vi "Helningsvinkel Demo.vi"() -> ()   [LabVIEW 2015]
doc: "Use this template to build a standard state machine design pattern. Each state executes code and determines which state to transition to. Contrast this design pattern with the User Interface Event Handler pattern, in which code executes in response to user actions. Contrast this design pattern also with the Queued Message Handler pattern, in which each message handling code can queue zero or more new messages."
panel:
  in  "Tab Control":T1(tab)
  in  "Senterområde \n[Grader]":dbl=10.0
  out "Horisontal":bool
  out "Calibrated Accelerations":waveform(dbl)[](graph)
  out "Helningsvinkel [Grader]":T2(graph)=[{[{"Tilt Angles [Deg][0]"=-0.6144374241661963, "Tilt Angles [Deg][1]"=86.381895519637}]}, {[{"Tilt Angles [Deg][0]"=44.252986428534086, "Tilt Angles [Deg][1]"=45.64924639869557}]}, {[{"Tilt Angles [Deg][0]"=-2.0, "Tilt Angles [Deg][1]"=-2.0}, {"Tilt Angles [Deg][0]"=-2.0, "Tilt Angles [Deg][1]"=2.0}, {"Tilt Angles [Deg][0]"=2.0, "Tilt Angles [Deg][1]"=2.0}, {"Tilt Angles [Deg][0]"=2.0, "Tilt Angles [Deg][1]"=-2.0}, {"Tilt Angles [Deg][0]"=-2.0, "Tilt Angles [Deg][1]"=-2.0}]}, {[{"Tilt Angles [Deg][0]"=90.0, "Tilt Angles [Deg][1]"=0.0}, {"Tilt Angles [Deg][0]"=87.16535433070865, "Tilt Angles [Deg][1]"=2.8346456692913384}, {"Tilt Angles [Deg][0]"=84.33070866141736, "Tilt Angles [Deg][1]"=5.669291338582677}, {"Tilt Angles [Deg][0]"=81.496062992126, "Tilt Angles [Deg][1]"=8.503937007874015}, {"Tilt Angles [Deg][0]"=78.66141732283465, "Tilt Angles [Deg][1]"=11.338582677165354}, {"Tilt Angles [Deg][0]"=75.8267716535433, "Tilt Angles [Deg][1]"=14.173228346456694}, {"Tilt Angles [Deg][0]"=72.99212598425198, "Tilt Angles [Deg][1]"=17.00787401574803}, {"Tilt Angles [Deg][0]"=70.15748031496065, "Tilt Angles [Deg][1]"=19.84251968503937}, {"Tilt Angles [Deg][0]"=67.3228346456693, "Tilt Angles [Deg][1]"=22.677165354330707}, {"Tilt Angles [Deg][0]"=64.48818897637794, "Tilt Angles [Deg][1]"=25.511811023622048}, {"Tilt Angles [Deg][0]"=61.65354330708662, "Tilt Angles [Deg][1]"=28.34645669291339}, {"Tilt Angles [Deg][0]"=58.818897637795274, "Tilt Angles [Deg][1]"=31.181102362204715}, {"Tilt Angles [Deg][0]"=55.98425196850394, "Tilt Angles [Deg][1]"=34.01574803149606}, {"Tilt Angles [Deg][0]"=53.14960629921261, "Tilt Angles [Deg][1]"=36.8503937007874}, {"Tilt Angles [Deg][0]"=50.314960629921266, "Tilt Angles [Deg][1]"=39.68503937007874}, {"Tilt Angles [Deg][0]"=47.480314960629926, "Tilt Angles [Deg][1]"=42.51968503937008}, {"Tilt Angles [Deg][0]"=44.645669291338585, "Tilt Angles [Deg][1]"=45.354330708661415}, {"Tilt Angles [Deg][0]"=41.81102362204725, "Tilt Angles [Deg][1]"=48.188976377952756}, {"Tilt Angles [Deg][0]"=38.97637795275591, "Tilt Angles [Deg][1]"=51.023622047244096}, {"Tilt Angles [Deg][0]"=36.14173228346457, "Tilt Angles [Deg][1]"=53.85826771653544}, {"Tilt Angles [Deg][0]"=33.30708661417323, "Tilt Angles [Deg][1]"=56.69291338582678}, {"Tilt Angles [Deg][0]"=30.472440944881885, "Tilt Angles [Deg][1]"=59.52755905511811}, {"Tilt Angles [Deg][0]"=27.637795275590555, "Tilt Angles [Deg][1]"=62.362204724409445}, {"Tilt Angles [Deg][0]"=24.80314960629921, "Tilt Angles [Deg][1]"=65.19685039370079}, {"Tilt Angles [Deg][0]"=21.968503937007878, "Tilt Angles [Deg][1]"=68.03149606299212}, {"Tilt Angles [Deg][0]"=19.133858267716533, "Tilt Angles [Deg][1]"=70.86614173228347}, {"Tilt Angles [Deg][0]"=16.2992125984252, "Tilt Angles [Deg][1]"=73.7007874015748}, {"Tilt Angles [Deg][0]"=13.464566929133856, "Tilt Angles [Deg][1]"=76.53543307086616}, {"Tilt Angles [Deg][0]"=10.629921259842522, "Tilt Angles [Deg][1]"=79.3700787401575}, {"Tilt Angles [Deg][0]"=7.795275590551192, "Tilt Angles [Deg][1]"=82.20472440944883}, {"Tilt Angles [Deg][0]"=4.960629921259845, "Tilt Angles [Deg][1]"=85.03937007874012}, {"Tilt Angles [Deg][0]"=2.1259842519685126, "Tilt Angles [Deg][1]"=87.8740157480315}, {"Tilt Angles [Deg][0]"=-0.7086614173228328, "Tilt Angles [Deg][1]"=89.29133858267735}, {"Tilt Angles [Deg][0]"=-3.5433070866141656, "Tilt Angles [Deg][1]"=86.45669291338587}, {"Tilt Angles [Deg][0]"=-6.377952755905511, "Tilt Angles [Deg][1]"=83.6220472440945}, {"Tilt Angles [Deg][0]"=-9.212598425196845, "Tilt Angles [Deg][1]"=80.78740157480318}, {"Tilt Angles [Deg][0]"=-12.047244094488189, "Tilt Angles [Deg][1]"=77.9527559055118}, {"Tilt Angles [Deg][0]"=-14.881889763779522, "Tilt Angles [Deg][1]"=75.11811023622049}, {"Tilt Angles [Deg][0]"=-17.716535433070867, "Tilt Angles [Deg][1]"=72.28346456692913}, {"Tilt Angles [Deg][0]"=-20.5511811023622, "Tilt Angles [Deg][1]"=69.4488188976378}, {"Tilt Angles [Deg][0]"=-23.385826771653544, "Tilt Angles [Deg][1]"=66.61417322834644}, {"Tilt Angles [Deg][0]"=-26.220472440944878, "Tilt Angles [Deg][1]"=63.77952755905513}, {"Tilt Angles [Deg][0]"=-29.05511811023622, "Tilt Angles [Deg][1]"=60.944881889763785}, {"Tilt Angles [Deg][0]"=-31.889763779527545, "Tilt Angles [Deg][1]"=58.110236220472466}, {"Tilt Angles [Deg][0]"=-34.72440944881888, "Tilt Angles [Deg][1]"=55.27559055118111}, {"Tilt Angles [Deg][0]"=-37.55905511811023, "Tilt Angles [Deg][1]"=52.44094488188977}, {"Tilt Angles [Deg][0]"=-40.393700787401585, "Tilt Angles [Deg][1]"=49.60629921259843}, {"Tilt Angles [Deg][0]"=-43.228346456692904, "Tilt Angles [Deg][1]"=46.7716535433071}, {"Tilt Angles [Deg][0]"=-46.062992125984245, "Tilt Angles [Deg][1]"=43.937007874015755}, {"Tilt Angles [Deg][0]"=-48.897637795275585, "Tilt Angles [Deg][1]"=41.102362204724415}, {"Tilt Angles [Deg][0]"=-51.73228346456693, "Tilt Angles [Deg][1]"=38.26771653543307}, {"Tilt Angles [Deg][0]"=-54.56692913385826, "Tilt Angles [Deg][1]"=35.43307086614175}, {"Tilt Angles [Deg][0]"=-57.40157480314961, "Tilt Angles [Deg][1]"=32.5984251968504}, {"Tilt Angles [Deg][0]"=-60.23622047244095, "Tilt Angles [Deg][1]"=29.763779527559056}, {"Tilt Angles [Deg][0]"=-63.070866141732296, "Tilt Angles [Deg][1]"=26.929133858267715}, {"Tilt Angles [Deg][0]"=-65.90551181102362, "Tilt Angles [Deg][1]"=24.094488188976392}, {"Tilt Angles [Deg][0]"=-68.74015748031495, "Tilt Angles [Deg][1]"=21.259842519685044}, {"Tilt Angles [Deg][0]"=-71.57480314960631, "Tilt Angles [Deg][1]"=18.4251968503937}, {"Tilt Angles [Deg][0]"=-74.40944881889763, "Tilt Angles [Deg][1]"=15.59055118110238}, {"Tilt Angles [Deg][0]"=-77.24409448818898, "Tilt Angles [Deg][1]"=12.755905511811035}, {"Tilt Angles [Deg][0]"=-80.0787401574803, "Tilt Angles [Deg][1]"=9.92125984251969}, {"Tilt Angles [Deg][0]"=-82.91338582677166, "Tilt Angles [Deg][1]"=7.0866141732283445}, {"Tilt Angles [Deg][0]"=-85.74803149606302, "Tilt Angles [Deg][1]"=4.251968503937025}, {"Tilt Angles [Deg][0]"=-88.58267716535435, "Tilt Angles [Deg][1]"=1.4173228346456799}, {"Tilt Angles [Deg][0]"=-88.58267716535435, "Tilt Angles [Deg][1]"=-1.4173228346456657}, {"Tilt Angles [Deg][0]"=-85.74803149606302, "Tilt Angles [Deg][1]"=-4.251968503937011}, {"Tilt Angles [Deg][0]"=-82.91338582677166, "Tilt Angles [Deg][1]"=-7.086614173228331}, {"Tilt Angles [Deg][0]"=-80.07874015748034, "Tilt Angles [Deg][1]"=-9.921259842519676}, {"Tilt Angles [Deg][0]"=-77.24409448818898, "Tilt Angles [Deg][1]"=-12.75590551181102}, {"Tilt Angles [Deg][0]"=-74.40944881889763, "Tilt Angles [Deg][1]"=-15.590551181102368}, {"Tilt Angles [Deg][0]"=-71.57480314960631, "Tilt Angles [Deg][1]"=-18.42519685039369}, {"Tilt Angles [Deg][0]"=-68.74015748031496, "Tilt Angles [Deg][1]"=-21.259842519685034}, {"Tilt Angles [Deg][0]"=-65.90551181102363, "Tilt Angles [Deg][1]"=-24.094488188976378}, {"Tilt Angles [Deg][0]"=-63.07086614173231, "Tilt Angles [Deg][1]"=-26.929133858267697}, {"Tilt Angles [Deg][0]"=-60.23622047244096, "Tilt Angles [Deg][1]"=-29.763779527559045}, {"Tilt Angles [Deg][0]"=-57.401574803149614, "Tilt Angles [Deg][1]"=-32.598425196850386}, {"Tilt Angles [Deg][0]"=-54.56692913385827, "Tilt Angles [Deg][1]"=-35.43307086614173}, {"Tilt Angles [Deg][0]"=-51.732283464566954, "Tilt Angles [Deg][1]"=-38.26771653543305}, {"Tilt Angles [Deg][0]"=-48.89763779527561, "Tilt Angles [Deg][1]"=-41.1023622047244}, {"Tilt Angles [Deg][0]"=-46.06299212598426, "Tilt Angles [Deg][1]"=-43.93700787401575}, {"Tilt Angles [Deg][0]"=-43.22834645669291, "Tilt Angles [Deg][1]"=-46.77165354330708}, {"Tilt Angles [Deg][0]"=-40.39370078740159, "Tilt Angles [Deg][1]"=-49.60629921259841}, {"Tilt Angles [Deg][0]"=-37.55905511811025, "Tilt Angles [Deg][1]"=-52.440944881889756}, {"Tilt Angles [Deg][0]"=-34.724409448818896, "Tilt Angles [Deg][1]"=-55.275590551181104}, {"Tilt Angles [Deg][0]"=-31.88976377952756, "Tilt Angles [Deg][1]"=-58.11023622047245}, {"Tilt Angles [Deg][0]"=-29.055118110236215, "Tilt Angles [Deg][1]"=-60.944881889763785}, {"Tilt Angles [Deg][0]"=-26.220472440944917, "Tilt Angles [Deg][1]"=-63.77952755905508}, {"Tilt Angles [Deg][0]"=-23.38582677165357, "Tilt Angles [Deg][1]"=-66.61417322834644}, {"Tilt Angles [Deg][0]"=-20.55118110236223, "Tilt Angles [Deg][1]"=-69.44881889763776}, {"Tilt Angles [Deg][0]"=-17.71653543307088, "Tilt Angles [Deg][1]"=-72.28346456692913}, {"Tilt Angles [Deg][0]"=-14.881889763779538, "Tilt Angles [Deg][1]"=-75.11811023622046}, {"Tilt Angles [Deg][0]"=-12.047244094488189, "Tilt Angles [Deg][1]"=-77.9527559055118}, {"Tilt Angles [Deg][0]"=-9.212598425196845, "Tilt Angles [Deg][1]"=-80.78740157480314}, {"Tilt Angles [Deg][0]"=-6.3779527559055005, "Tilt Angles [Deg][1]"=-83.6220472440945}, {"Tilt Angles [Deg][0]"=-3.543307086614205, "Tilt Angles [Deg][1]"=-86.45669291338577}, {"Tilt Angles [Deg][0]"=-0.7086614173228596, "Tilt Angles [Deg][1]"=-89.29133858267735}, {"Tilt Angles [Deg][0]"=2.125984251968486, "Tilt Angles [Deg][1]"=-87.8740157480315}, {"Tilt Angles [Deg][0]"=4.96062992125983, "Tilt Angles [Deg][1]"=-85.03937007874019}, {"Tilt Angles [Deg][0]"=7.795275590551176, "Tilt Angles [Deg][1]"=-82.20472440944883}, {"Tilt Angles [Deg][0]"=10.629921259842522, "Tilt Angles [Deg][1]"=-79.3700787401575}, {"Tilt Angles [Deg][0]"=13.464566929133868, "Tilt Angles [Deg][1]"=-76.53543307086613}, {"Tilt Angles [Deg][0]"=16.299212598425164, "Tilt Angles [Deg][1]"=-73.70078740157484}, {"Tilt Angles [Deg][0]"=19.133858267716505, "Tilt Angles [Deg][1]"=-70.8661417322835}, {"Tilt Angles [Deg][0]"=21.968503937007853, "Tilt Angles [Deg][1]"=-68.03149606299215}, {"Tilt Angles [Deg][0]"=24.803149606299197, "Tilt Angles [Deg][1]"=-65.1968503937008}, {"Tilt Angles [Deg][0]"=27.63779527559054, "Tilt Angles [Deg][1]"=-62.36220472440946}, {"Tilt Angles [Deg][0]"=30.472440944881885, "Tilt Angles [Deg][1]"=-59.52755905511811}, {"Tilt Angles [Deg][0]"=33.30708661417324, "Tilt Angles [Deg][1]"=-56.69291338582678}, {"Tilt Angles [Deg][0]"=36.14173228346458, "Tilt Angles [Deg][1]"=-53.85826771653543}, {"Tilt Angles [Deg][0]"=38.976377952755875, "Tilt Angles [Deg][1]"=-51.023622047244125}, {"Tilt Angles [Deg][0]"=41.811023622047216, "Tilt Angles [Deg][1]"=-48.18897637795279}, {"Tilt Angles [Deg][0]"=44.645669291338564, "Tilt Angles [Deg][1]"=-45.35433070866144}, {"Tilt Angles [Deg][0]"=47.480314960629904, "Tilt Angles [Deg][1]"=-42.519685039370096}, {"Tilt Angles [Deg][0]"=50.31496062992125, "Tilt Angles [Deg][1]"=-39.685039370078755}, {"Tilt Angles [Deg][0]"=53.1496062992126, "Tilt Angles [Deg][1]"=-36.8503937007874}, {"Tilt Angles [Deg][0]"=55.98425196850395, "Tilt Angles [Deg][1]"=-34.01574803149605}, {"Tilt Angles [Deg][0]"=58.81889763779525, "Tilt Angles [Deg][1]"=-31.18110236220476}, {"Tilt Angles [Deg][0]"=61.653543307086586, "Tilt Angles [Deg][1]"=-28.346456692913417}, {"Tilt Angles [Deg][0]"=64.48818897637793, "Tilt Angles [Deg][1]"=-25.511811023622073}, {"Tilt Angles [Deg][0]"=67.32283464566927, "Tilt Angles [Deg][1]"=-22.67716535433073}, {"Tilt Angles [Deg][0]"=70.15748031496062, "Tilt Angles [Deg][1]"=-19.84251968503938}, {"Tilt Angles [Deg][0]"=72.99212598425198, "Tilt Angles [Deg][1]"=-17.007874015748037}, {"Tilt Angles [Deg][0]"=75.82677165354332, "Tilt Angles [Deg][1]"=-14.17322834645669}, {"Tilt Angles [Deg][0]"=78.66141732283465, "Tilt Angles [Deg][1]"=-11.338582677165345}, {"Tilt Angles [Deg][0]"=81.49606299212596, "Tilt Angles [Deg][1]"=-8.50393700787405}, {"Tilt Angles [Deg][0]"=84.33070866141729, "Tilt Angles [Deg][1]"=-5.669291338582704}, {"Tilt Angles [Deg][0]"=87.16535433070865, "Tilt Angles [Deg][1]"=-2.8346456692913593}, {"Tilt Angles [Deg][0]"=90.0, "Tilt Angles [Deg][1]"=-1.4033418597069752e-14}]}]
  # "Helningsmåling med akselerometer"
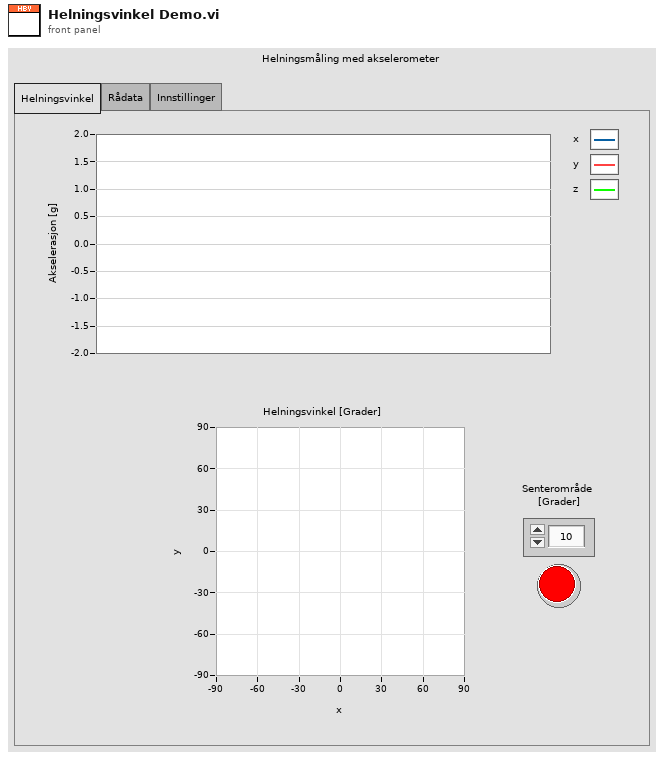
[diagram p1: front panel]
types:
  T1 = enum32{"Helningsvinkel", "Rådata", "Innstillinger"}
  T2 = cluster{cluster{"Tilt Angles [Deg][0]":dbl, "Tilt Angles [Deg][1]":dbl}[]}[]
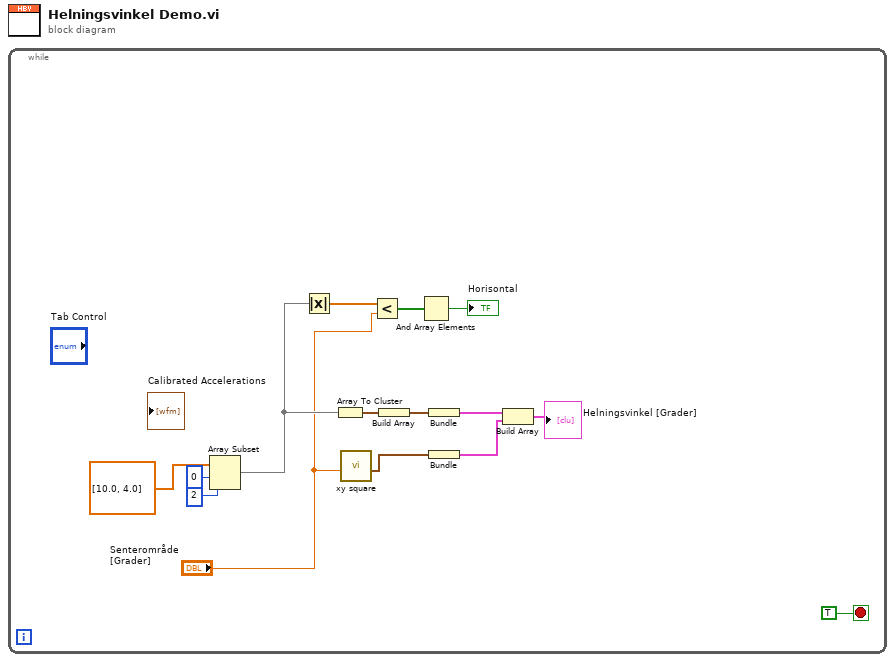
[diagram p0: block diagram]
diagram:
  n1 = while {
    stop <- TRUE stop-if-true
    n2 = Array Subset(array=dbl[] [10.0, 4.0], index=0, length=2) -> (w6:dbl[])
    n3 = Absolute Value(x=w6) -> (abs(x)=w14:dbl[])
    n4 = Array To Cluster(array=w6) -> (cluster=w15:cluster{"[0]":dbl, "[1]":dbl})
    n5 = call "xy square.vi"("Side"="Senterområde \n[Grader]") -> ("xy Data"=w2:cluster{"x":dbl, "y":dbl}[])  [unwired: 9 in, 1 out]
    n6 = Less?(x=w14, y="Senterområde \n[Grader]") -> (x < y?=w10:bool[])
    n7 = Build Array(w15) -> (w12:cluster{"[0]":dbl, "[1]":dbl}[])
    n8 = And Array Elements(Boolean array=w10) -> (logical AND=→"Horisontal":bool)
    n9 = Bundle(w12) -> (w11:cluster{cluster{"[0]":dbl, "[1]":dbl}[]})  [unwired: 1 in]
    n10 = Bundle("xy Data"=w2) -> (w3:cluster{"xy Data":cluster{"x":dbl, "y":dbl}[]})  [unwired: 1 in]
    n11 = Build Array(w11, w3) -> (→"Helningsvinkel [Grader]":cluster{"xy Data":cluster{"x":dbl, "y":dbl}[]}[])
  }
